vi "Example Callback.vi"() -> ()   [LabVIEW 2010]
uses:
  C:/tf/play/labview/Tinkerforge.dll
  Tinkerforge.dll
panel:
  in  "stop":bool
  in  "uid":string="63oL6P"
  in  "port":i32=4223
  in  "host":string="localhost"
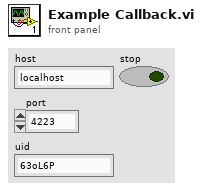
[diagram p1: front panel]
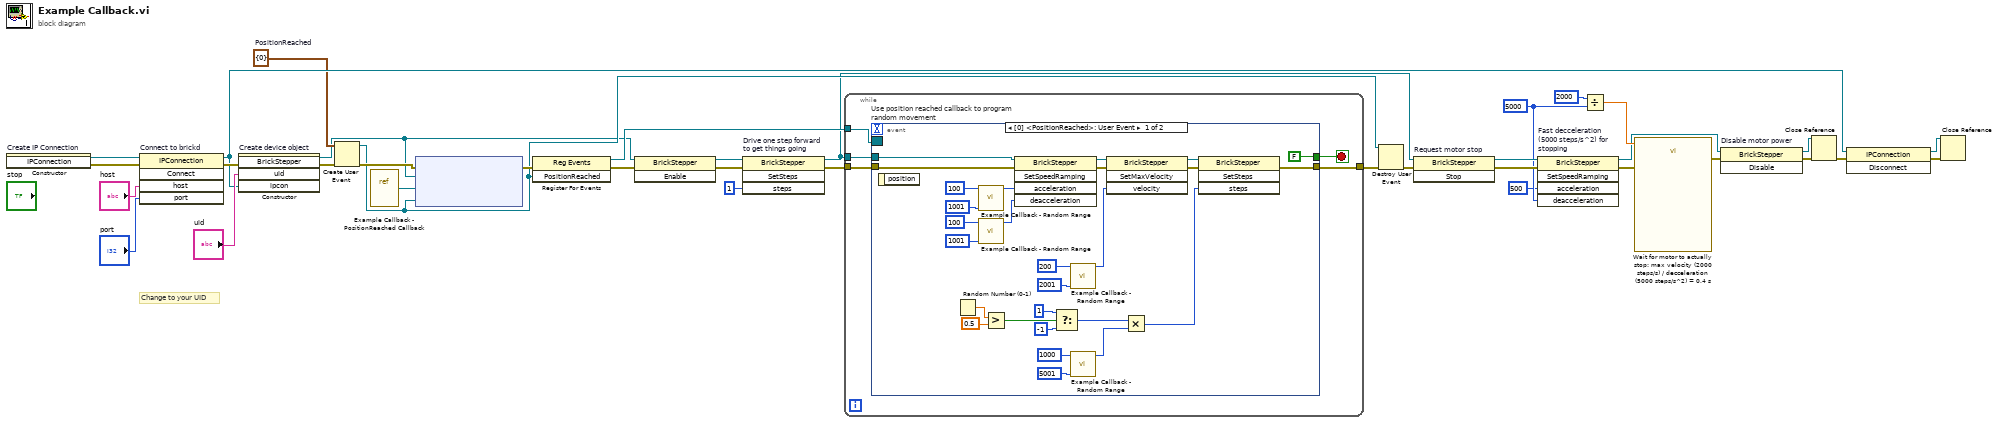
[diagram p0: block diagram]
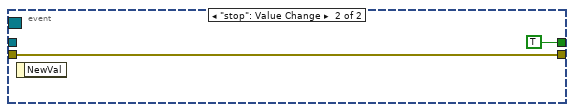
[diagram p2: hidden frame]
diagram:
  w7 = 5000 ("deacceleration")
  w23 = cluster{"position":i32} {"position"=0}  # PositionReached
  # "Change to your UID"
  n1 = constructor on="Create IP Connection" class="IPConnection"() -> (reference out=w37:refnum<k24>, error out=w14:errorcluster)  [unwired: 3 in, 1 out]
  n2 = invoke on="Connect to brickd" class="IPConnection" method="Connect"(reference=w37, error in=w14, "host"="host", "port"="port") -> (reference out=w30:refnum<k24>, error out=w33:errorcluster)  [unwired: 1 in, 3 out]
  n3 = constructor on="Create device object" class="BrickStepper"(error in=w33, "uid"="uid", "ipcon"=w30) -> (reference out=w20:refnum<k24>, error out=w22:errorcluster)  [unwired: 2 in, 3 out]
  n4 = Create User Event(user event datatype=w23, error in=w22) -> (user event=w24:refnum<user-event>, error out=w28:errorcluster)
  n5 = vi-ref "Example Callback - PositionReached Callback.vi"() -> ("vi reference"=w15:refnum<vi>)
  n6 = node ("Register Event Callback")(w28, w20, w15, w24) -> (w27:errorcluster)  [unwired: 1 in, 1 out]
  n7 = register-events(error in=w27, w24) -> (reference out=w26:refnum<event-registration>, error out=w19:errorcluster)  [unwired: 1 in]
  n8 = invoke class="BrickStepper" method="Enable"(reference=w20, error in=w19) -> (reference out=w21:refnum<k24>, error out=w18:errorcluster)  [unwired: 1 in, 1 out]
  n9 = invoke on="Drive one step forward\nto get things going" class="BrickStepper" method="SetSteps"(reference=w21, error in=w18, "steps"=1) -> (reference out=w4:refnum<k24>, error out=w17:errorcluster)  [unwired: 1 in, 2 out]
  n10 = while {
    tunnel: w26 -> [w42]
    tunnel: [w41] -> w25
    tunnel: w17 -> [w40]
    tunnel: w4 -> [w39]
    stop <- w38 stop-if-true
    n11 = event "Use position reached callback to program random movement" shown="[0] <PositionReached>: User Event" {
      selector: w42 -> [_ _]
      dyn-events: _ -> [_ _]
      timeout: _ -> [_ _]
      tunnel: [w69 w70] -> w41
      tunnel: w40 -> [w65 w70]
      tunnel: w39 -> [w44 _]
      tunnel: [FALSE TRUE] -> w38
      event User Event {
        n12 = event-data() -> ()  [unwired: 1 in, 1 out]
        n13 = Random Number (0-1)() -> (number: 0 to 1=w52:dbl)
        n14 = call "Example Callback - Random Range.vi"("max"=1001, "min"=100) -> ("random"=w63:i32)  [unwired: 9 in]
        n15 = call "Example Callback - Random Range.vi"("max"=1001, "min"=100) -> ("random"=w62:i32)  [unwired: 9 in]
        n16 = Greater?(x=w52, y=0.5) -> (0:w50:bool)
        n17 = invoke class="BrickStepper" method="SetSpeedRamping"(reference=w44, error in=w65, "acceleration"=w63, "deacceleration"=w62) -> (reference out=w66:refnum<k24>, error out=w64:errorcluster)  [unwired: 1 in, 3 out]
        n18 = Select(t=1, s=w50, f=-1) -> (s? t:f=w47:i32)
        n19 = call "Example Callback - Random Range.vi"("max"=2001, "min"=200) -> ("random"=w57:i32)  [unwired: 9 in]
        n20 = call "Example Callback - Random Range.vi"("max"=5001, "min"=1000) -> ("random"=w46:i32)  [unwired: 9 in]
        n21 = invoke class="BrickStepper" method="SetMaxVelocity"(reference=w66, error in=w64, "velocity"=w57) -> (reference out=w68:refnum<k24>, error out=w67:errorcluster)  [unwired: 1 in, 2 out]
        n22 = Multiply(x=w47, y=w46) -> (x*y=w45:i32)
        n23 = invoke class="BrickStepper" method="SetSteps"(reference=w68, error in=w67, "steps"=w45) -> (error out=w69:errorcluster)  [unwired: 1 in, 3 out]
      }
      event "stop": Value Change {
        n24 = event-data() -> ()  [unwired: 1 in, 1 out]
      }
    }
  }
  n25 = Destroy User Event(user event=w24, error in=w25) -> (error out=w5:errorcluster)
  n26 = invoke on="Request motor stop" class="BrickStepper" method="Stop"(reference=w4, error in=w5) -> (reference out=w11:refnum<k24>, error out=w9:errorcluster)  [unwired: 1 in, 1 out]
  n27 = invoke on="Fast decceleration\n(5000 steps/s^2) for\nstopping" class="BrickStepper" method="SetSpeedRamping"(reference=w11, error in=w9, "acceleration"=500, "deacceleration"=w7) -> (reference out=w10:refnum<k24>, error out=w8:errorcluster)  [unwired: 1 in, 3 out]
  n28 = Divide(x=2000, y=w7) -> (x/y=w12:dbl)
  n29 = call "Wait for motor to actually stop: max velocity (2000 steps/s) / decceleration (5000 steps/s^2) = 0.4 s"("error in (no error)"=w8, "Delay Time (s)"=w12) -> ("error out"=w13:errorcluster)  [unwired: 9 in]
  n30 = invoke on="Disable motor power" class="BrickStepper" method="Disable"(reference=w10, error in=w13) -> (reference out=w2:refnum<k24>, error out=w3:errorcluster)  [unwired: 1 in, 1 out]
  n31 = Close Reference(reference=w2, error in (no error)=w3) -> (error out=w32:errorcluster)
  n32 = invoke class="IPConnection" method="Disconnect"(reference=w30, error in=w32) -> (reference out=w29:refnum<k24>, error out=w31:errorcluster)  [unwired: 1 in, 1 out]
  n33 = Close Reference(reference=w29, error in (no error)=w31) -> ()  [unwired: 1 out]
